vi "Shoot.vi"(10 "Shoot?":bool, 11 "Set RPM":dbl) -> ()   [LabVIEW 2016]
uses:
  <vilib>/gmath/NI_Gmath.lvlib
panel:
  in  "OR Speed":dbl=1.0
  in  "Override?":bool
  in  "RPM Array":dbl[](array[numeric]) format="%_6g"
  in  "Control":dbl[](array[numeric]) format="%_6g"
  in  "kP":dbl
  out "Shooter RPM":dbl
  out "Shooter RPM":dbl
  out "Encoder Index Count":dbl format="%#_13g"
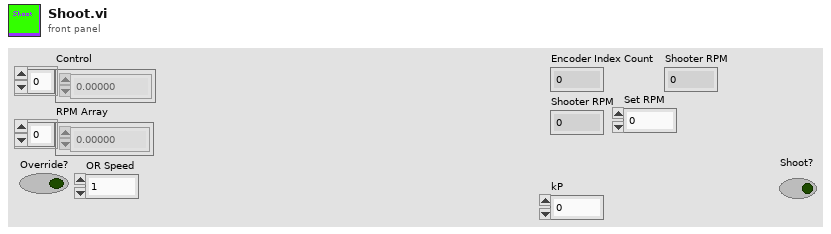
[diagram p1: front panel]
types:
  T1 = typedef "WPI_MotorControlDeviceRef.ctl" = cluster{"DeviceStatus":errorcluster, "Type":T2, "PWM":cluster{"PWM Channel":T3, "DeadBand":T4}, "CAN":cluster{"Device Number":u8, "SetOutput VI Ref":variant, "GetOutput VI Ref":variant, "Enable VI Ref":variant, "Disable VI Ref":variant, "Data":variant}, "Invert":bool}
  T2 = typedef "WPI_MotorControlType.ctl" = enum16{"PWM", "CAN"}
  T3 = typedef "FPGA_DIOPWMChannel.ctl" = enum8{"PWM 0", "PWM 1", "PWM 2", "PWM 3", "PWM 4", "PWM 5", "PWM 6", "PWM 7", "PWM 8", "PWM 9", "PWM MXP 0", "PWM MXP 1", "PWM MXP 2", "PWM MXP 3", "PWM MXP 4", "PWM MXP 5", "PWM MXP 6", "PWM MXP 7", "PWM MXP 8", "PWM MXP 9", "Invalid"}
  T4 = typedef "WPI_PWMDeadband.ctl" = cluster{"Name":string, "maxPositivePwm":i32, "minPositivePwm":i32, "centerPwm":i32, "maxNegativePwm":i32, "minNegativePwm":i32, "angularRange":u16}
  T5 = typedef "WPI_CANTalonSRX_GlobalStatus.ctl" = cluster{"Applied Throttle":dbl, "Module Enabled":bool, "CAN Error":errorcluster, "Closed Loop Error":dbl, "Forward Limit Switch Closed":bool, "Reverse Limit Switch Closed":bool, "Sensor Position":dbl, "Sensor Velocity":dbl, "Current":dbl, "Sticky Fault - Over Temp":bool, "Sticky Fault - Under Voltage":bool, "Sticky Fault - Forward Limit":bool, "Sticky Fault - Reverse Limit":bool, "Sticky Fault - Forward Soft Limit":bool, "Sticky Fault - Reverse Soft Limit":bool, "Brake is Enabled":bool, "Encoder Position":dbl, "Encoder Velocity":dbl, "Encoder Index Count":dbl, "Encoder A Pin State":bool, "Encoder B Pin State":bool, "Encoder Index Pin State":bool, "Analog In":dbl, "Analog In Velocity":dbl, "Temperature (C)":dbl, "Battery Voltage":dbl, "Control 5 Is Supported":bool, "Current Profile Slot Select":dbl, "Pos Div 8":bool, "Vel Div 4":bool, "Pulse Width Position":i32, "Pulse Width Velocity":i32, "Pulse Width Rise To Rise (us)":i32, "Pulse Width Rise To Fall (us)":i32, "Mot Prof Active Is Under Run":bool, "Mot Prof Active Has Under Run":bool, "Mot Prof Active Is Last":bool, "Mot Prof Active Velocity Only":bool, "Mot Prof Active Is Valid":bool, "Mot Prof Buffer Is Full":bool, "Mot Prof Active Profile Slot Select":i32, "Mot Prof NextID":i32, "Mot Prof Count":i32, "Mot Prof Active Velocity":dbl, "Mot Prof Active Position":dbl, "Mot Prof Output Enable":i32}
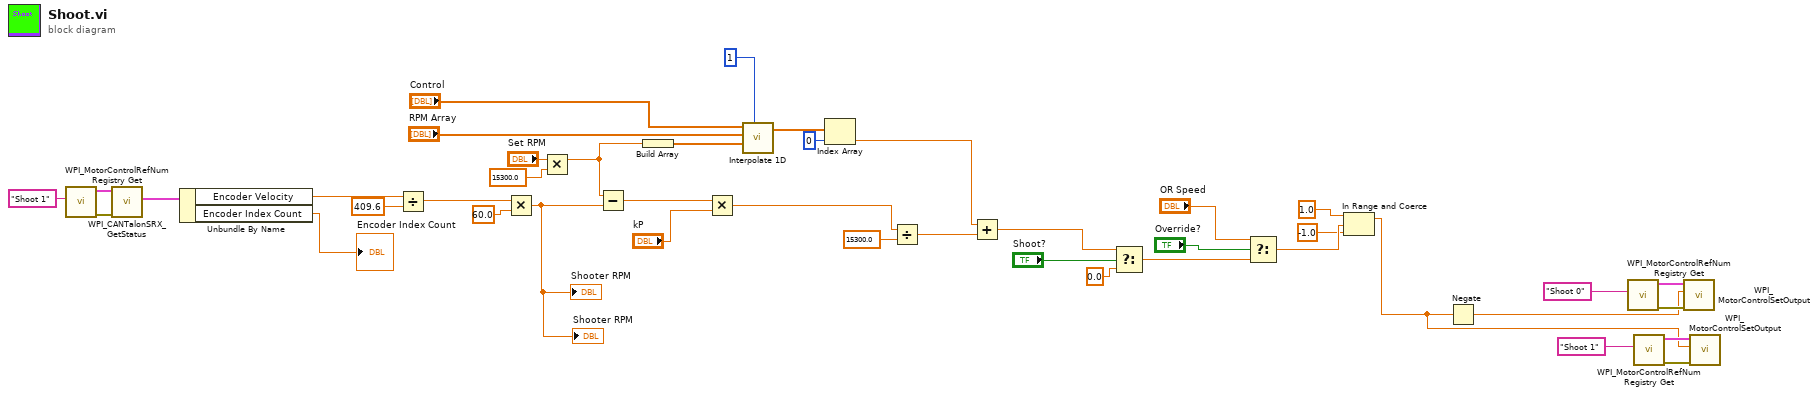
[diagram p0: block diagram]
diagram:
  n1 = call <vilib>:"WPI_MotorControlRefNum Registry Get.vi"("refnum name"="Shoot 1") -> ("error out"=w35:errorcluster, "MotorControlDevRef"=w34:T1)  [unwired: 9 in]
  n2 = call <vilib>:"WPI_CANTalonSRX_GetStatus.vi"("error in (no error)"=w35, "CAN Talon SRX Ref"=w34) -> ("Talon SRX Status"=w33:T5)  [unwired: 7 in, 2 out]
  n3 = Unbundle By Name(w33) -> ("Encoder Velocity"=w31:dbl, "Encoder Index Count"=→"Encoder Index Count":dbl)
  n4 = Divide(x=w31, y=409.6) -> (x/y=w29:dbl)
  n5 = Multiply(x=w29, y=60.0) -> (x*y=w27:dbl)
  "Shooter RPM" <- w27
  "Shooter RPM" <- w27
  n6 = Multiply(x="Set RPM", y=15300.0) -> (x*y=w4:dbl)
  n7 = Subtract(x=w4, y=w27) -> (x-y=w23:dbl)
  n8 = Build Array(w4) -> (w21:dbl[])
  n9 = Multiply(x=w23, y="kP") -> (x*y=w17:dbl)
  n10 = call <vilib>:"Interpolate 1D.vi"("method"=1, "xi"=w21, "X"="RPM Array", "Y"="Control") -> ("yi"=w25:dbl[])  [unwired: 5 in, 2 out]
  n11 = Index Array(array=w25, index=0) -> (element=w14:dbl)
  n12 = Divide(x=w17, y=15300.0) -> (x/y=w15:dbl)
  n13 = Add(x=w14, y=w15) -> (x+y=w13:dbl)
  n14 = Select(t=w13, s="Shoot?", f=0.0) -> (s? t:f=w11:dbl)
  n15 = Select(t="OR Speed", s="Override?", f=w11) -> (s? t:f=w8:dbl)
  n16 = In Range and Coerce(upper limit=1.0, x=w8, lower limit=-1.0) -> (coerced(x)=w1:dbl)  [unwired: 1 out]
  n17 = Negate(x=w1) -> (-x=w2:dbl)
  n18 = call <vilib>:"WPI_MotorControlRefNum Registry Get.vi"("refnum name"="Shoot 0") -> ("error out"=w40:errorcluster, "MotorControlDevRef"=w38:T1)  [unwired: 9 in]
  n19 = call <vilib>:"WPI_MotorControlRefNum Registry Get.vi"("refnum name"="Shoot 1") -> ("error out"=w37:errorcluster, "MotorControlDevRef"=w41:T1)  [unwired: 9 in]
  n20 = call <vilib>:"WPI_MotorControlSetOutput.vi"("error in (no error)"=w40, "Output"=w2, "MotorControlDevRef"=w38) -> ()  [unwired: 6 in, 3 out]
  n21 = call <vilib>:"WPI_MotorControlSetOutput.vi"("error in (no error)"=w37, "Output"=w1, "MotorControlDevRef"=w41) -> ()  [unwired: 6 in, 3 out]
